vi "SetGetLEDStripRef.vi"(8 "error in":errorcluster, 10 "Enum":enum16{"get", "set"}(ring), 11 "LEDStripRef in":T1={"PWM Rate (Hz)"=1000.0, "Max Duty Cycle"=1000.0, "DigitalOutputRed"={"Digital Module"=enum."Digital Module 1", "DIO Channel"=enum."DIO 1", "DevStatus"={"status"=FALSE, "code"=0, "source"=""}}, "DigitalOutputGreen"={"Digital Module"=enum."Digital Module 1", "DIO Channel"=enum."DIO 1", "DevStatus"={"status"=FALSE, "code"=0, "source"=""}}, "DigitalOutputBlue"={"Digital Module"=enum."Digital Module 1", "DIO Channel"=enum."DIO 1", "DevStatus"={"status"=FALSE, "code"=0, "source"=""}}, "DevStatus"={"status"=FALSE, "code"=0, "source"=""}}) -> (0 "error out":errorcluster, 3 "LEDStripRef out":T1={"PWM Rate (Hz)"=1000.0, "Max Duty Cycle"=1000.0, "DigitalOutputRed"={"Digital Module"=enum."Digital Module 1", "DIO Channel"=enum."DIO 1", "DevStatus"={"status"=FALSE, "code"=0, "source"=""}}, "DigitalOutputGreen"={"Digital Module"=enum."Digital Module 1", "DIO Channel"=enum."DIO 1", "DevStatus"={"status"=FALSE, "code"=0, "source"=""}}, "DigitalOutputBlue"={"Digital Module"=enum."Digital Module 1", "DIO Channel"=enum."DIO 1", "DevStatus"={"status"=FALSE, "code"=0, "source"=""}}, "DevStatus"={"status"=FALSE, "code"=0, "source"=""}})   [LabVIEW 2014]
uses:
  LEDStripRef.ctl
  <vilib>/Rock Robotics/WPI/DigitalOutput/WPI_DigitalOutputDevRef.ctl
  <vilib>/Rock Robotics/SystemInterfaces/Typedef/FPGA_TypedefDigitalModule.ctl
  <vilib>/Rock Robotics/SystemInterfaces/DIO/FPGA_DIOChannel.ctl
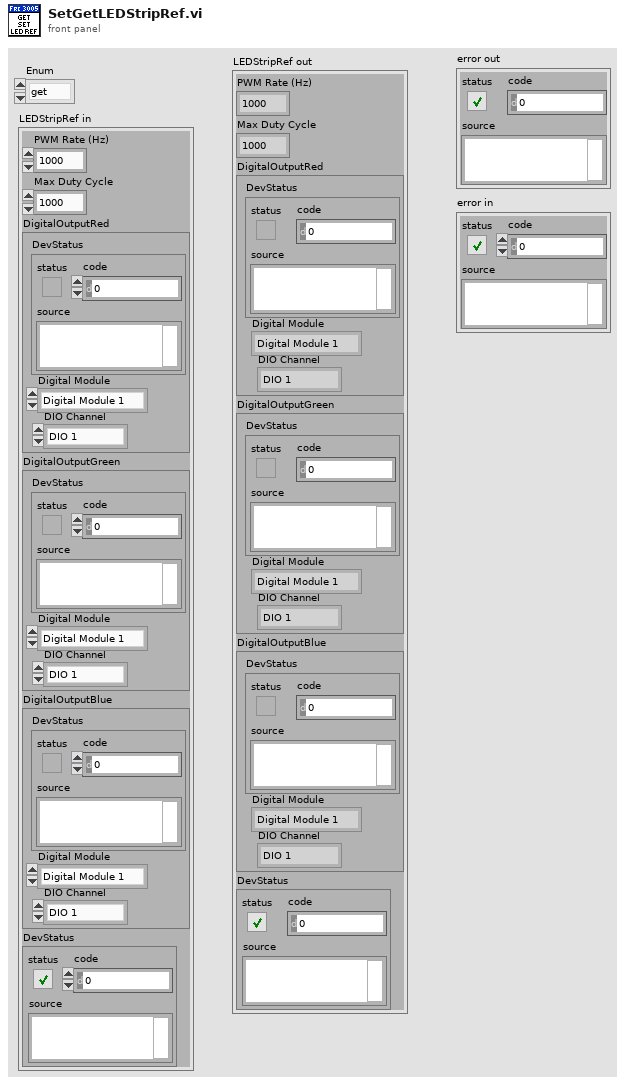
[diagram p1: front panel]
types:
  T1 = typedef "LEDStripRef.ctl" = cluster{"PWM Rate (Hz)":sgl, "Max Duty Cycle":sgl, "DigitalOutputRed":T2, "DigitalOutputGreen":T2, "DigitalOutputBlue":T2, "DevStatus":errorcluster}
  T2 = typedef "WPI_DigitalOutputDevRef.ctl" = cluster{"Digital Module":T3, "DIO Channel":T4, "DevStatus":errorcluster}
  T3 = typedef "FPGA_TypedefDigitalModule.ctl" = enum16{"Digital Module 1", "Digital Module 2"}
  T4 = typedef "FPGA_DIOChannel.ctl" = enum8{"DIO 1", "DIO 2", "DIO 3", "DIO 4", "DIO 5", "DIO 6", "DIO 7", "DIO 8", "DIO 9", "DIO 10", "DIO 11", "DIO 12", "DIO 13", "DIO 14", "Invalid"}
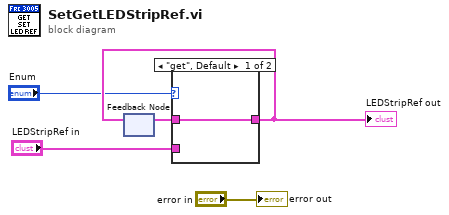
[diagram p0: block diagram]
diagram:
  n1 = feedback #1() -> (w5:T1)  [unwired: 1 in]
  n2 = case shown="\"get\", Default" "Enum" {
    tunnel: "LEDStripRef in" -> [_ w7]
    tunnel: [w6 w7] -> w4
    tunnel: w5 -> [w6 _]
    frame "get", Default {
    }
    frame "set" {
    }
  }
  "LEDStripRef out" <- w4
  n3 = feedback-in #1(w4) -> ()
  "error out" <- "error in"
